vi "FTW-Reflection-FTWObject.vi"(7 "FTWObject Type":variant) -> (8 "FTW Object Type":string)   [LabVIEW 2015]
panel:
  # "Inputs"
  # "Outputs"
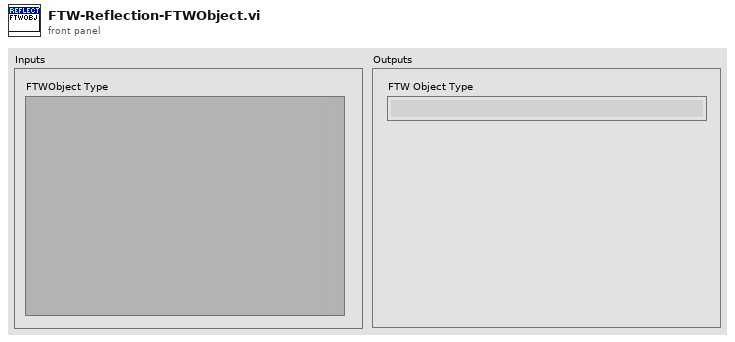
[diagram p1: front panel]
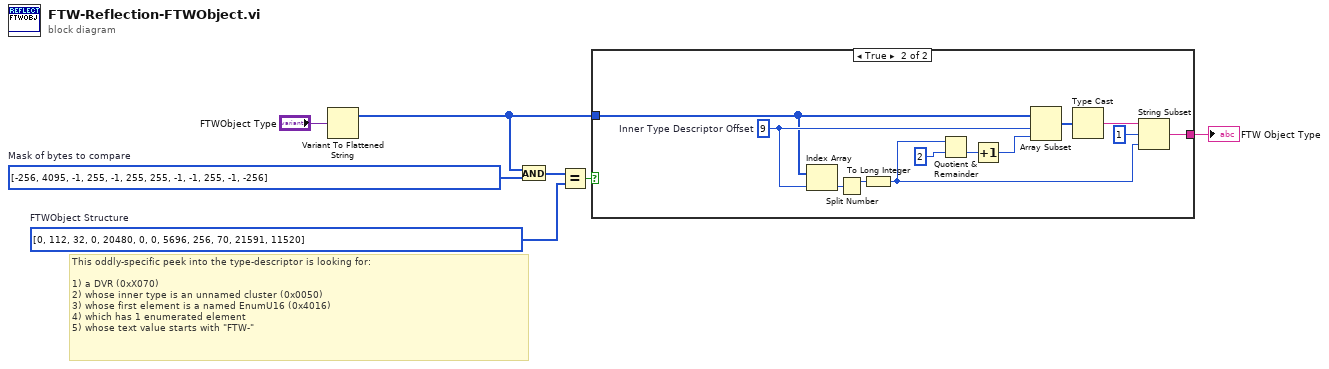
[diagram p0: block diagram]
diagram:
  w2 = i16[] [0, 112, 32, 0, 20480, 0, 0, 5696, 256, 70, 21591, 11520]  # FTWObject Structure
  w4 = i16[] [-256, 4095, -1, 255, -1, 255, 255, -1, -1, 255, -1, -256]  # Mask of bytes to compare
  # "This oddly-specific peek into the type-descriptor is looking for:\n\n1) a DVR (0xX070)\n2) whose inner type is an unnamed cluster (0x0050)\n3) whose first element is a named EnumU16 (0x4016)\n4) which has 1 enumerated element\n5) whose text value starts with \"FTW-\""
  n1 = Variant To Flattened String(Variant="FTWObject Type") -> (1:w5:i16[])  [unwired: 1 out]
  n2 = And(x=w5, y=w4) -> (x .and. y?=w3:i16[])
  n3 = Equal?(x=w3, y=w2) -> (x = y?=w1:bool)
  n4 = case shown="True" w1 {
    tunnel: w5 -> [_ w17]
    tunnel: [_ w8] -> w6
    frame False {
    }
    frame True {
      w18 = 9  # Inner Type Descriptor Offset
      n5 = Index Array(array=w17, index=w18) -> (element=w16:i16)
      n6 = Split Number(x=w16) -> (hi(x)=w15:u8)  [unwired: 1 out]
      n7 = To Long Integer(number=w15) -> (32bit integer=w10:i32)
      n8 = Quotient & Remainder(x=w10, y=2) -> (floor(x/y)=w13:i32)  [unwired: 1 out]
      n9 = Increment(x=w13) -> (x+1=w12:i32)
      n10 = Array Subset(array=w17, index=w18, length=w12) -> (w14:i16[])
      n11 = Type Cast(x=w14) -> (*(type *) &x=w9:string)  [unwired: 1 in]
      n12 = String Subset(string=w9, offset (0)=1, length (rest)=w10) -> (substring=w8:string)
    }
  }
  "FTW Object Type" <- w6
